vi "SR201_init.vi"(8 "error in":errorcluster, 10 "port":u16=6722, 11 "address":string="192.168.24.184") -> (0 "error out":errorcluster, 1 "ch2":bool, 2 "ch1":bool, 3 "conn_id":refnum<k5>, 4 "status":bool)   [LabVIEW 2019]
panel:
  out "state":string
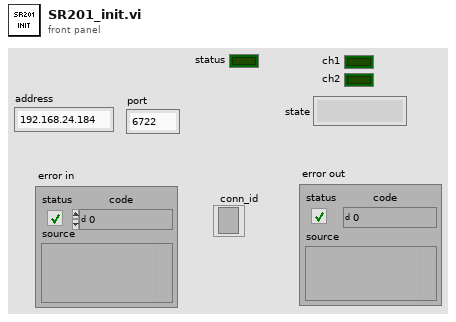
[diagram p1: front panel]
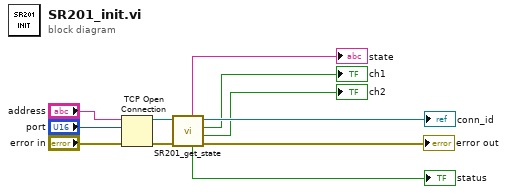
[diagram p0: block diagram]
diagram:
  n1 = TCP Open Connection(address="address", remote port or service name="port", error in (no error)="error in") -> (connection ID=w8:refnum<k5>, error out=w7:errorcluster)  [unwired: 2 in]
  n2 = call "SR201_get_state.vi"("error in"=w7, "conn_id_in"=w8) -> ("error out"=→"error out":errorcluster, "ch2"=→"ch2":bool, "ch1"=→"ch1":bool, "conn_id_out"=→"conn_id":refnum<k5>, "status"=→"status":bool, "string"=→"state":string)  [unwired: 4 in]
